vi "T7_Read_UINT16_Register.vi"(6 "Num Registers to read":i32=2, 8 "error in (no error)":errorcluster, 9 "FirstChannel":i32, 11 "Remote IP Address":string="192.168.126.148") -> (0 "error out":errorcluster, 1 "LastRead":timestamp=timestamp(3513857842.218402 s since 1904-01-01), 2 "Read UINT16":u16, 3 "Raw Data Read":u16[](array[numeric]))   [LabVIEW 2018]
uses:
  <vilib>/Plasmionique/MB Master/MB_Master_TCP/MB_Master_TCP.lvclass
  Applications/National Instruments/LabVIEW 2018 64-bit/vi.lib/Plasmionique/MB Master/MB_Master/MB_Master.lvclass
  <vilib>/Plasmionique/MB Master/MB Master.lvlib
panel:
  out "Array":dbl[](array[numeric])
  out "LastValue":dbl
  # "MB Ethernet Example Master.vi\n\nInstructions\n1.Use Kipling to find your devices IP address & modify the\n\"Remote IP Addres\"\n2. Run this VI\n3. Change value of \"UINT16 to Write\" & press \"Write Data\""
  # "TCP Parameters"
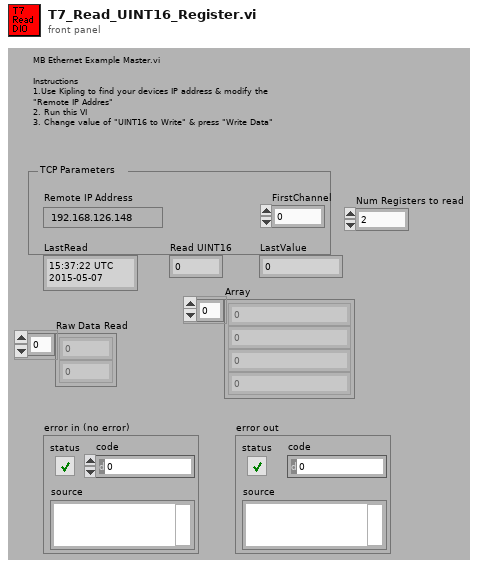
[diagram p1: front panel]
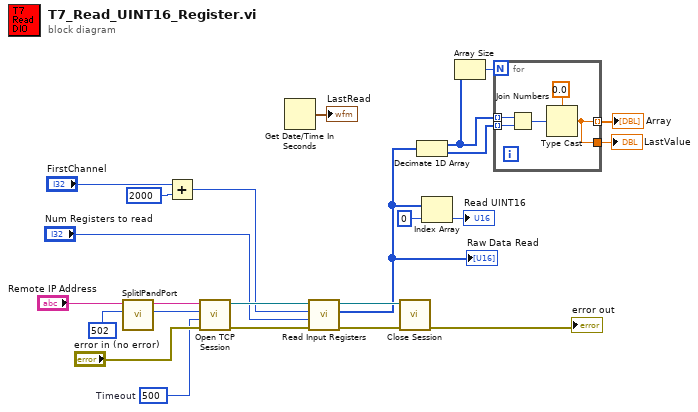
[diagram p0: block diagram]
diagram:
  w7 = 500  # Timeout
  n1 = call "SplitIPandPort.vi"("defaultPort(10001)"=u16 502, "IP:Port"="Remote IP Address") -> ("Port"=w1:u16, "IP"=w4:string)  [unwired: 8 in]
  n2 = Add(x="FirstChannel", y=2000) -> (x+y=w6:i32)
  n3 = call <vilib>:"Open TCP Session.vi"("error in (no error)"="error in (no error)", "Timeout (10000)"=w7, "Port (502)"=w1, "IP Address"=w4) -> ("error out"=w23:errorcluster, "MB_TCP session"=w24:refnum<class "MB_Master_TCP.lvclass">)  [unwired: 6 in]
  n4 = Get Date/Time In Seconds() -> (seconds since 1Jan1904=→"LastRead":timestamp)
  n5 = call <vilib>:"Read Input Registers.vi"("error in (no error)"=w23, "quantity"="Num Registers to read", "starting address"=w6, "MB session in"=w24) -> ("error out"=w22:errorcluster, "Registers"=w11:u16[], "MB session out"=w21:refnum<class "MB_Master_TCP.lvclass">)  [unwired: 5 in]
  "Raw Data Read" <- w11
  n6 = call-dynamic "Close Session.vi"("error in (no error)"=w22, "MB TCP session"=w21) -> ("error out"=→"error out":errorcluster)  [unwired: 9 in]
  n7 = Decimate 1D Array(w11) -> (w13:u16[], w14:u16[])
  n8 = Index Array(array=w11, index=0) -> (element=→"Read UINT16":u16)
  n9 = Array Size(array=w13) -> (size(s)=w12:i32)
  n10 = for {
    N: w12 -> [_]
    tunnel: w13 -> [w28] mode=indexing
    tunnel: w14 -> [w29] mode=indexing
    tunnel: [w25] -> w15 mode=indexing
    tunnel: [w25] -> w16
    n11 = Join Numbers(hi=w28, lo=w29) -> ((hi.lo)=w27:u32)
    n12 = Type Cast(type=sgl 0.0, x=w27) -> (*(type *) &x=w25:sgl)
  }
  "Array" <- w15
  "LastValue" <- w16
